vi "Calcu_Force Weight.vi"(4 "기준기 데이터":string[][](array[string]), 7 "방향":string, 8 "분해능":string, 10 "Condition":string[][](array[string]), 11 "분동조합":string[][](array[string])) -> (0 "Condition Out":string[][](array[string]), 1 "에러 배열":bool[](array[boolean]), 2 "사용기준추":string[][](array[string]), 3 "기준추 데이터":string[][](array[string]))   [LabVIEW 2020]
uses:
  Public/Polymorph/Rmv Empt Arr_1D Str.vi
panel:
  out "배열":string[](array[string])
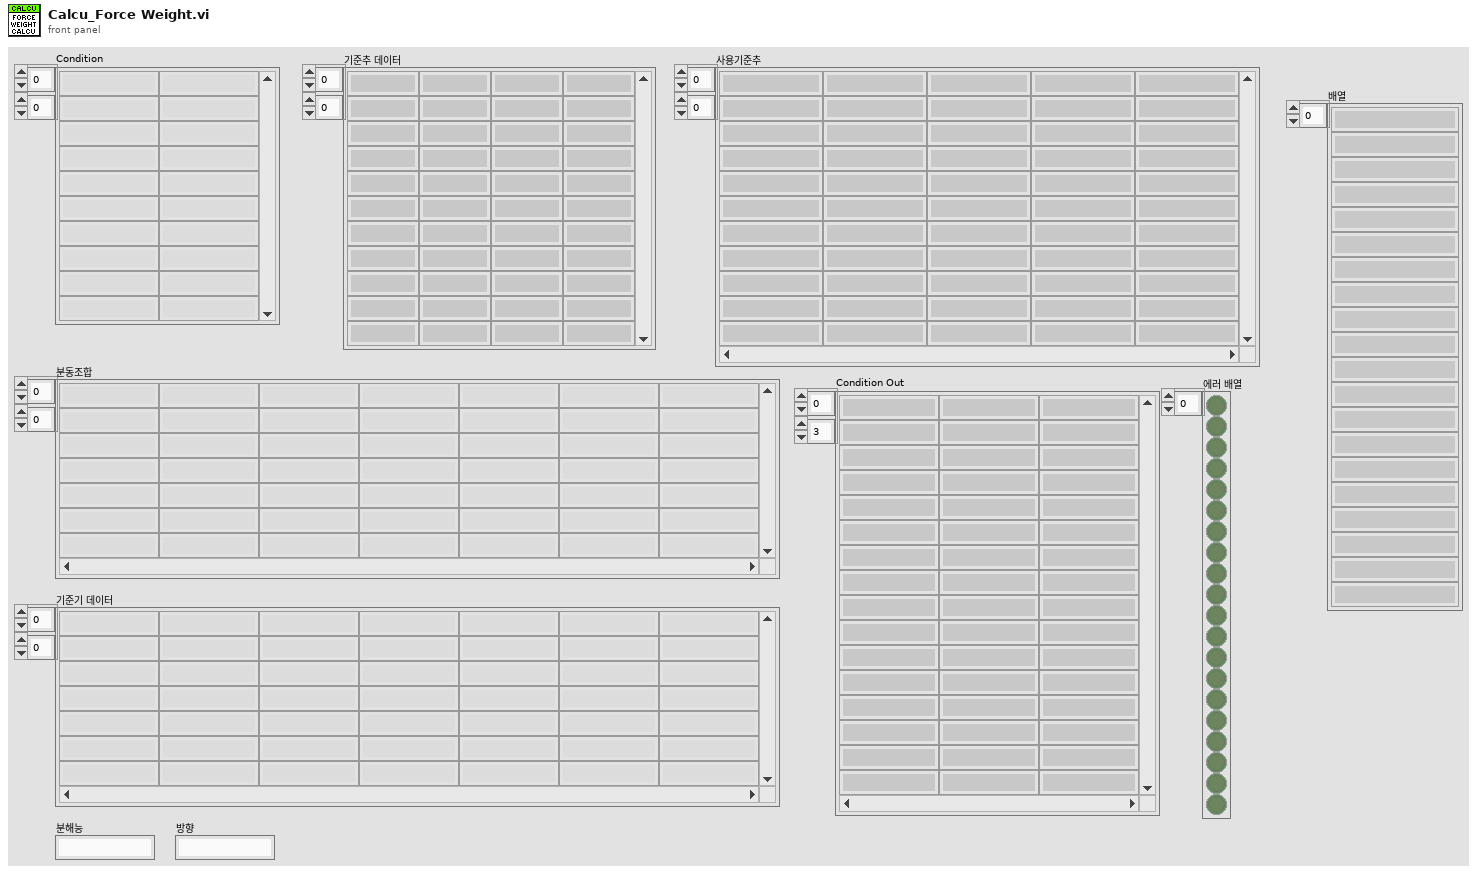
[diagram p1: front panel]
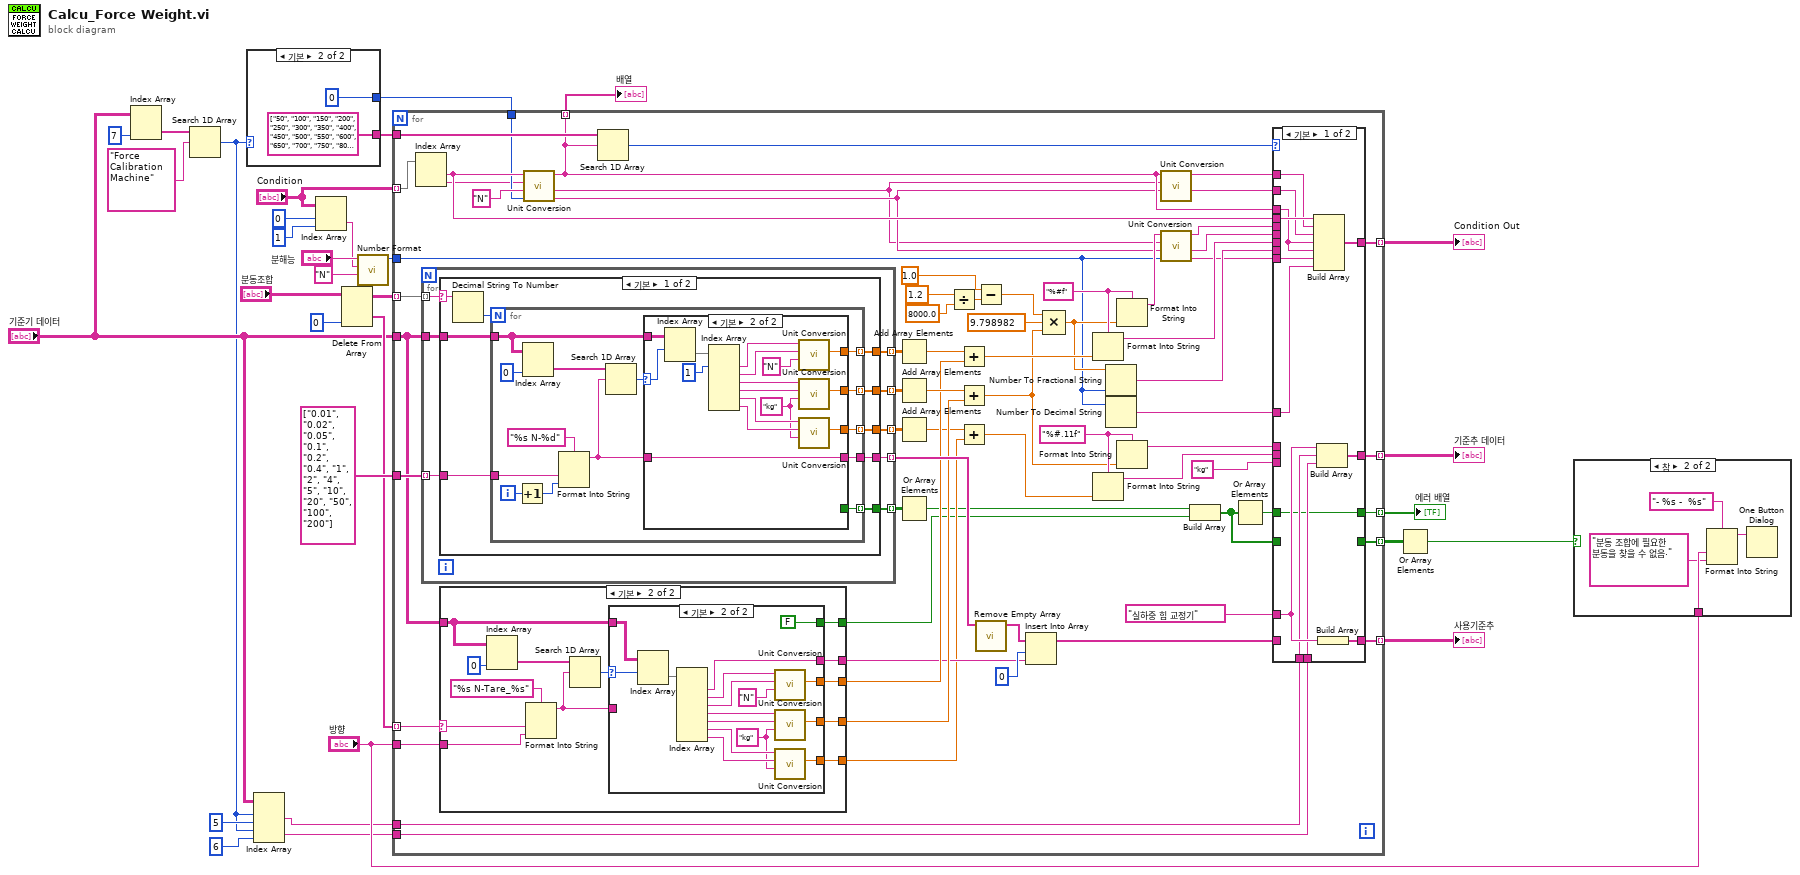
[diagram p0: block diagram]
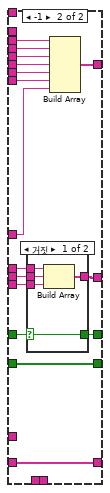
[diagram p4: hidden frame]
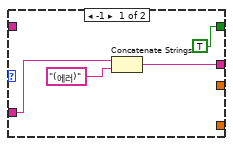
[diagram p7: hidden frame]
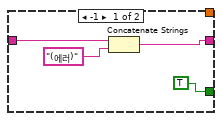
[diagram p8: hidden frame]
diagram:
  n1 = Index Array(array="기준기 데이터", index (col)=7 ("비활성화된 인덱스 (열)")) -> (element=w13:string[])  [unwired: 1 in]
  n2 = Search 1D Array(1D array=w13, element="Force Calibration Machine" ("원소")) -> (index of element=w8:i32)  [unwired: 1 in]
  n3 = case shown="기본" w8 {
    selector: w8 -> [w32 _]
    tunnel: [_ string[] ["50", "100", "150", "200", "250", "300", "350", "400", "450", "500", "550", "600", "650", "700", "750", "800", "850", "900", "950", "1000", "1050", "1100", "1150", "1200", "1250", "1300", "1350", "1400", "1450", "1500", "1550", "1600", "1650", "1700", "1750", "1800", "1850", "1900", "1950", "2000", "2050", "2100", "2150", "2200", "2250", "2300", "2350", "2400", "2450", "2500", "2550", "2600", "2650", "2700", "2750", "2800", "2850", "2900", "2950", "3000", "3050", "3100", "3150", "3200", "3250", "3300", "3350", "3400", "3450", "3500", "3550", "3600", "3650", "3700", "3750", "3800", "3850", "3900", "3950", "4000", "4050", "4100", "4150", "4200", "4250", "4300", "4350", "4400", "4450", "4500", "4550", "4600", "4650", "4700", "4750", "4800", "4850", "4900", "4950", "5000"] ("배열 2")] -> w15
    tunnel: [w32 0] -> w1
    frame -1 {
    }
    frame Default {
    }
  }
  n4 = Index Array(array="기준기 데이터", index (row) #1=w8, index (col) #1=5 ("비활성화된 인덱스 (열)"), index (row) #2=w8, index (col) #2=6 ("비활성화된 인덱스 (열)")) -> (element #1=w9:string, element #2=w6:string)
  n5 = Index Array(array="Condition", index (row)=0 ("인덱스 (행)"), index (col)=1 ("비활성화된 인덱스 (열)")) -> (element=w19:string)
  n6 = Delete From Array(array="분동조합", index (col)=0 ("비활성화된 인덱스 (열)")) -> (deleted portion=w26:string[], array with subset deleted=w29:string[][])  [unwired: 2 in]
  n7 = call "Number Format.vi"("기준단위"="N", "입력단위"=w19, "입력값"="분해능") -> ("정밀도(단위적용)"=w22:i32)  [unwired: 8 in]
  n8 = for {
    tunnel: w29 -> [w101] mode=indexing
    tunnel: string[] ["0.01", "0.02", "0.05", "0.1", "0.2", "0.4", "1", "2", "4", "5", "10", "20", "50", "100", "200"] -> [w100]
    tunnel: [w67] -> w27 mode=indexing
    tunnel: "기준기 데이터" -> [w90]
    tunnel: w26 -> [w82] mode=indexing
    tunnel: "방향" -> [w97]
    tunnel: "Condition" -> [w81] mode=indexing
    tunnel: w22 -> [w46]
    tunnel: [w68] -> w24 mode=indexing
    tunnel: [w69] -> w5 mode=indexing
    tunnel: [w77] -> w23 mode=indexing
    tunnel: w15 -> [w78]
    tunnel: w9 -> [w58]
    tunnel: w6 -> [w57]
    tunnel: [w51] -> w3 mode=indexing
    tunnel: [w47] -> w2 mode=indexing
    tunnel: w1 -> [w50]
    w83 = "%#.11f" ("포맷 문자열")
    w79 = "%#f" ("포맷 문자열")
    n9 = Index Array(array=w81) -> (element #1=w72:string, element #2=w45:string)  [unwired: 2 in]
    n10 = for {
      tunnel: w101 -> [w177] mode=indexing
      tunnel: w100 -> [w176] mode=indexing
      tunnel: [w175] -> w94 mode=indexing
      tunnel: w90 -> [w174]
      tunnel: [w173] -> w99 mode=indexing
      tunnel: [w172] -> w96 mode=indexing
      tunnel: [w171] -> w91 mode=indexing
      tunnel: [w170] -> w52 mode=indexing
      n11 = case shown="기본" w177 {
        selector: w177 -> [w186 _]
        tunnel: w176 -> [w184 _]
        tunnel: [w183 _] -> w175
        tunnel: w174 -> [w182 _]
        tunnel: [w181 _] -> w173
        tunnel: [w180 _] -> w172
        tunnel: [w179 _] -> w171
        tunnel: [w178 _] -> w170
        frame Default {
          n12 = Decimal String To Number(string=w186) -> (number=w185:i32)  [unwired: 2 in, 1 out]
          n13 = for {
            N: w185 -> [_]
            tunnel: w184 -> [w200]
            tunnel: [w188] -> w183
            tunnel: w182 -> [w194]
            tunnel: [w193] -> w181 mode=indexing
            tunnel: [w192] -> w180 mode=indexing
            tunnel: [w191] -> w179 mode=indexing
            tunnel: [w189] -> w178 mode=indexing
            i -> [w198]
            n14 = Increment(x=w198) -> (x+1=w197:i32)
            n15 = Index Array(array=w194, index (col)=0 ("비활성화된 인덱스 (열)")) -> (element=w195:string[])  [unwired: 1 in]
            n16 = Format Into String(format string="%s N-%d" ("포맷 문자열"), w200, w197) -> (resulting string=w187:string)  [unwired: 2 in, 1 out]
            n17 = Search 1D Array(1D array=w195, element=w187) -> (index of element=w190:i32)  [unwired: 1 in]
            n18 = case shown="기본" w190 {
              selector: w190 -> [_ w206]
              tunnel: w194 -> [_ w220]
              tunnel: [_ w214] -> w193
              tunnel: [_ w211] -> w192
              tunnel: [_ w207] -> w191
              tunnel: [TRUE _] -> w189
              tunnel: [w201 w205] -> w188
              tunnel: w187 -> [w202 w205]
              frame -1 {
                n19 = Concatenate Strings(w202, "(에러)" ("문자열")) -> (w201:string)
              }
              frame Default {
                w208 = "kg" ("환산단위")
                n20 = Index Array(array=w220, index (row)=w206) -> (element=w219:string[])  [unwired: 1 in]
                n21 = Index Array(array=w219, index #1=1 ("인덱스")) -> (element #1=w217:string, element #2=w216:string, element #3=w213:string, element #4=w212:string, element #5=w210:string, element #6=w209:string)  [unwired: 5 in]
                n22 = call "Unit Conversion.vi"("환산단위"="N", "입력단위"=w216, "입력값"=w217) -> ("환산값 (DBL)"=w214:dbl)  [unwired: 3 in, 5 out]
                n23 = call "Unit Conversion.vi"("환산단위"=w208, "입력단위"=w212, "입력값"=w213) -> ("환산값 (DBL)"=w211:dbl)  [unwired: 3 in, 5 out]
                n24 = call "Unit Conversion.vi"("환산단위"=w208, "입력단위"=w209, "입력값"=w210) -> ("환산값 (DBL)"=w207:dbl)  [unwired: 3 in, 5 out]
              }
            }
          }
        }
        frame "" {
        }
      }
    }
    n25 = case shown="기본" w82 {
      selector: w82 -> [_ w139]
      tunnel: w97 -> [_ w147]
      tunnel: w90 -> [_ w146]
      tunnel: [_ w144] -> w89
      tunnel: [_ w143] -> w88
      tunnel: [_ w142] -> w87
      tunnel: [_ w141] -> w84
      tunnel: [_ w140] -> w54
      frame "" {
      }
      frame Default {
        n26 = Index Array(array=w146, index (col)=0 ("비활성화된 인덱스 (열)")) -> (element=w149:string[])  [unwired: 1 in]
        n27 = Format Into String(format string="%s N-Tare_%s" ("포맷 문자열"), w139, w147) -> (resulting string=w137:string)  [unwired: 2 in, 1 out]
        n28 = Search 1D Array(1D array=w149, element=w137) -> (index of element=w145:i32)  [unwired: 1 in]
        n29 = case shown="기본" w145 {
          selector: w145 -> [_ w156]
          tunnel: w146 -> [_ w169]
          tunnel: [_ w164] -> w144
          tunnel: [_ w161] -> w143
          tunnel: [_ w157] -> w141
          tunnel: [TRUE FALSE] -> w140
          tunnel: [w151 w154] -> w142
          tunnel: w137 -> [w152 _]
          frame -1 {
            n30 = Concatenate Strings(w152, "(에러)" ("문자열")) -> (w151:string)
          }
          frame Default {
            w158 = "kg" ("환산단위")
            n31 = Index Array(array=w169, index (row)=w156) -> (element=w168:string[])  [unwired: 1 in]
            n32 = Index Array(array=w168) -> (element #1=w154:string, element #2=w167:string, element #3=w166:string, element #4=w163:string, element #5=w162:string, element #6=w160:string, element #7=w159:string)  [unwired: 7 in]
            n33 = call "Unit Conversion.vi"("환산단위"="N", "입력단위"=w166, "입력값"=w167) -> ("환산값 (DBL)"=w164:dbl)  [unwired: 3 in, 5 out]
            n34 = call "Unit Conversion.vi"("환산단위"=w158, "입력단위"=w162, "입력값"=w163) -> ("환산값 (DBL)"=w161:dbl)  [unwired: 3 in, 5 out]
            n35 = call "Unit Conversion.vi"("환산단위"=w158, "입력단위"=w159, "입력값"=w160) -> ("환산값 (DBL)"=w157:dbl)  [unwired: 3 in, 5 out]
          }
        }
      }
    }
    n36 = call "Unit Conversion.vi"("소수점 자리수"=w50, "환산단위"="N", "입력단위"=w45, "입력값"=w72) -> ("입력단위"=w44:string, "환산단위"=w43:string, "환산값 (string)"=w47:string)  [unwired: 2 in, 3 out]
    n37 = Search 1D Array(1D array=w78, element=w47) -> (index of element=w70:i32)  [unwired: 1 in]
    n38 = Add Array Elements(numeric array=w99) -> (sum=w98:dbl)
    n39 = Add Array Elements(numeric array=w96) -> (sum=w95:dbl)
    n40 = Add Array Elements(numeric array=w91) -> (sum=w86:dbl)
    n41 = Or Array Elements(Boolean array=w52) -> (logical OR=w53:bool)
    n42 = Divide(x=1.2, y=8000.0) -> (x/y=w39:dbl)
    n43 = Add(x=w98, y=w89) -> (x+y=w80:dbl)
    n44 = Add(x=w95, y=w88) -> (x+y=w40:dbl)
    n45 = Add(x=w86, y=w84) -> (x+y=w85:dbl)
    n46 = Subtract(x=1.0, y=w39) -> (x-y=w35:dbl)
    n47 = call-poly "Remove Empty Array.vi"("Data in"=w94) -> ("Data out"=w93:string[])  [unwired: 9 in, 1 out]
    n48 = Insert Into Array(array=w93, index=0 ("인덱스"), new element=w87) -> (w66:string[])
    n49 = Compound Arithmetic op=MULTIPLY(w35, 9.798982 ("x"), w40) -> (w61:dbl)
    n50 = Format Into String(format string=w79, w80) -> (resulting string=w74:string)  [unwired: 2 in, 1 out]
    n51 = Format Into String(format string=w83, w85) -> (resulting string=w64:string)  [unwired: 2 in, 1 out]
    n52 = Number To Fractional String(number=w61, precision (6)=w46) -> (F-format string=w73:string)  [unwired: 2 in]
    n53 = Number To Decimal String(number=w46) -> (decimal integer string=w60:string)  [unwired: 1 in]
    n54 = Format Into String(format string=w79, w61) -> (resulting string=w56:string)  [unwired: 2 in, 1 out]
    n55 = Format Into String(format string=w83, w40) -> (resulting string=w65:string)  [unwired: 2 in, 1 out]
    n56 = call "Unit Conversion.vi"("환산단위"=w44, "입력단위"=w43, "입력값"=w47) -> ("환산단위"=w48:string, "환산값 (string)"=w49:string)  [unwired: 3 in, 4 out]
    n57 = call "Unit Conversion.vi"("소수점 자리수"=w46, "환산단위"=w44, "입력단위"=w43, "입력값"=w56) -> ("입력단위"=w42:string, "환산단위"=w75:string, "환산값 (string)"=w76:string)  [unwired: 2 in, 3 out]
    n58 = Build Array(w53, w54) -> (w55:bool[])
    n59 = Or Array Elements(Boolean array=w55) -> (logical OR=w62:bool)
    n60 = case shown="기본" w70 {
      tunnel: [w114 w130] -> w77
      tunnel: w72 -> [w106 w129]
      tunnel: w76 -> [_ w128]
      tunnel: w75 -> [_ w127]
      tunnel: w74 -> [_ w126]
      tunnel: w73 -> [_ w125]
      tunnel: w42 -> [w105 w124]
      tunnel: [_ w123] -> w69
      tunnel: w55 -> [_ w123]
      tunnel: [w113 w117] -> w68
      tunnel: [w111 w122] -> w67
      tunnel: w66 -> [_ w122]
      tunnel: w65 -> [_ w121]
      tunnel: w64 -> [_ w120]
      tunnel: "kg" ("환산단위") -> [_ w119]
      tunnel: w62 -> [w107 w118]
      tunnel: w60 -> [w108 w116]
      tunnel: "실하중 힘 교정기" -> [w112 _]
      tunnel: w58 -> [w110 _]
      tunnel: w57 -> [w109 _]
      tunnel: [w107 w115] -> w51
      tunnel: w49 -> [w103 _]
      tunnel: w48 -> [w104 _]
      tunnel: w47 -> [w102 _]
      frame Default {
        n61 = Build Array(w106, w103, w104, w102, w102, w105, w108) -> (w114:string[])
        n62 = Build Array(w112, w110, w109) -> (w113:string[])
        n63 = Build Array(w112) -> (w111:string[])
      }
      frame -1 {
        n64 = case shown="거짓" w118 {
          selector: w118 -> [w131 w136]
          tunnel: [w135 _] -> w117
          tunnel: w119 -> [w134 _]
          tunnel: w121 -> [w133 _]
          tunnel: w120 -> [w132 _]
          tunnel: [w131 w136] -> w115
          frame False {
            n65 = Build Array(w133, w132, w134) -> (w135:string[])
          }
          frame True {
          }
        }
        n66 = Build Array(w129, w128, w127, w126, w125, w124, w116) -> (w130:string[])
      }
    }
  }
  "사용기준추" <- w27
  "Condition Out" <- w23
  "기준추 데이터" <- w24
  "에러 배열" <- w3
  "배열" <- w2
  n67 = Or Array Elements(Boolean array=w5) -> (logical OR=w4:bool)
  n68 = case shown="참" w4 {
    tunnel: "방향" -> [_ w224]
    frame False {
    }
    frame True {
      n69 = Format Into String(format string="- %s -  %s" ("포맷 문자열"), w224, "분동 조합에 필요한 분동을 찾을 수 없음." ("메시지")) -> (resulting string=w222:string)  [unwired: 2 in, 1 out]
      n70 = One Button Dialog(message=w222) -> ()  [unwired: 1 in, 1 out]
    }
  }
